vi "repmat.vi"(9 "number of repeats":dbl, 11 "element":dbl) -> (3 "Array":dbl[](array[numeric]))   [LabVIEW 2017]
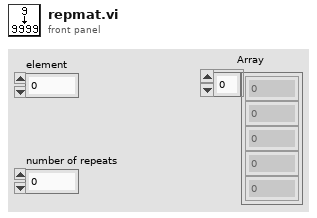
[diagram p1: front panel]
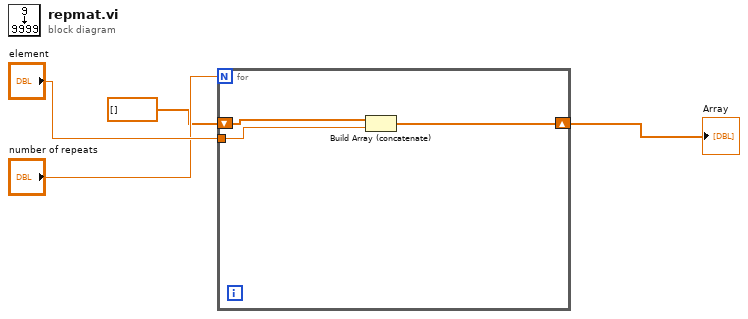
[diagram p0: block diagram]
diagram:
  n1 = for {
    N: "number of repeats" -> [_]
    tunnel: "element" -> [w5]
    shift-right: [w7] -> w2
    shift-left: dbl[] [] -> [w6]
    n2 = Build Array (concatenate)(w6, w5) -> (w7:dbl[])
  }
  "Array" <- w2
